vi "Subida.vi"(8 "thetaf":dbl, 10 "thetai":dbl) -> (2 "dt":dbl)   [LabVIEW 2018]
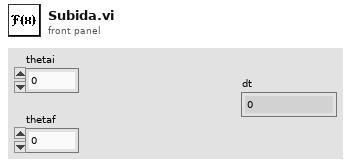
[diagram p1: front panel]
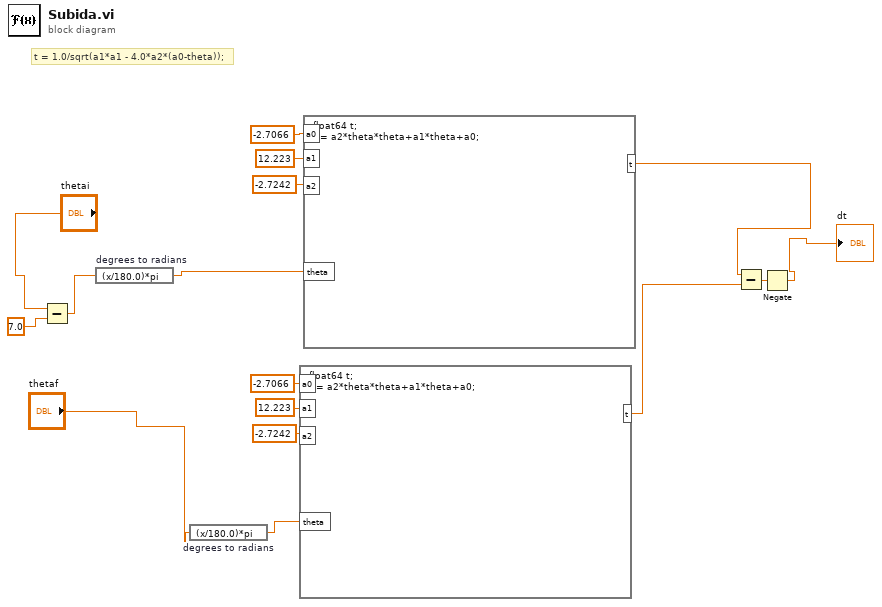
[diagram p0: block diagram]
diagram:
  # "t = 1.0/sqrt(a1*a1 - 4.0*a2*(a0-theta));"
  n1 = Subtract(x="thetai", y=7.0) -> (x-y=w3:dbl)
  n2 = expression code="(x/180.0)*pi" "degrees to radians"(w3) -> (w13:dbl)
  n3 = expression code="(x/180.0)*pi" "degrees to radians"("thetaf") -> (w5:dbl)
  n4 = formula code="float64 t;\nt = a2*theta*theta+a1*theta+a0;"("a0"=-2.7066 ("input variable"), "a1"=12.223 ("input variable"), "a2"=-2.7242 ("input variable"), "theta"=w5) -> ("t"=w4:dbl)
  n5 = formula code="float64 t;\nt = a2*theta*theta+a1*theta+a0;"("a0"=-2.7066 ("input variable"), "a1"=12.223 ("input variable"), "a2"=-2.7242 ("input variable"), "theta"=w13) -> ("t"=w11:dbl)
  n6 = Subtract(x=w11, y=w4) -> (x-y=w10:dbl)
  n7 = Negate(x=w10) -> (-x=→"dt":dbl)
